vi "Auto-Write to Folder and file for FEC_YCC.vi"(0 "Current PD (mV)":dbl, 4 "Centering data?":bool, 5 "Record Mode \npath(1,2)":bool[](array[boolean]), 6 "data to be saved":dbl[][](array[numeric]) format="%0.2f", 7 "Who's Data":enum16{"YCC", "PYW", "LCH", "YYH"}(ring), 8 "File name add to the end \n(height)":string="h300", 9 "Save?":bool) -> (2 "Save to File Name":string, 3 "Save to Path":path)   [LabVIEW 2014]
uses:
  Main-Stage-PI/(Global) Current handle and LaserPower_YCC.vi
  <vilib>/Utility/file.llb/Write To Spreadsheet File (DBL).vi
panel:
  out "Folder name":string
  out "folder exists?":bool
  out "date/time string":string
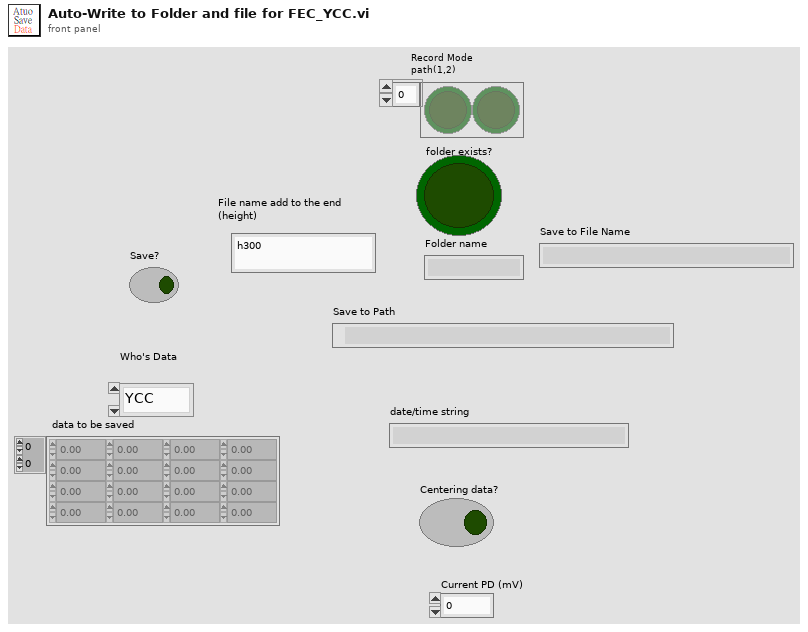
[diagram p1: front panel]
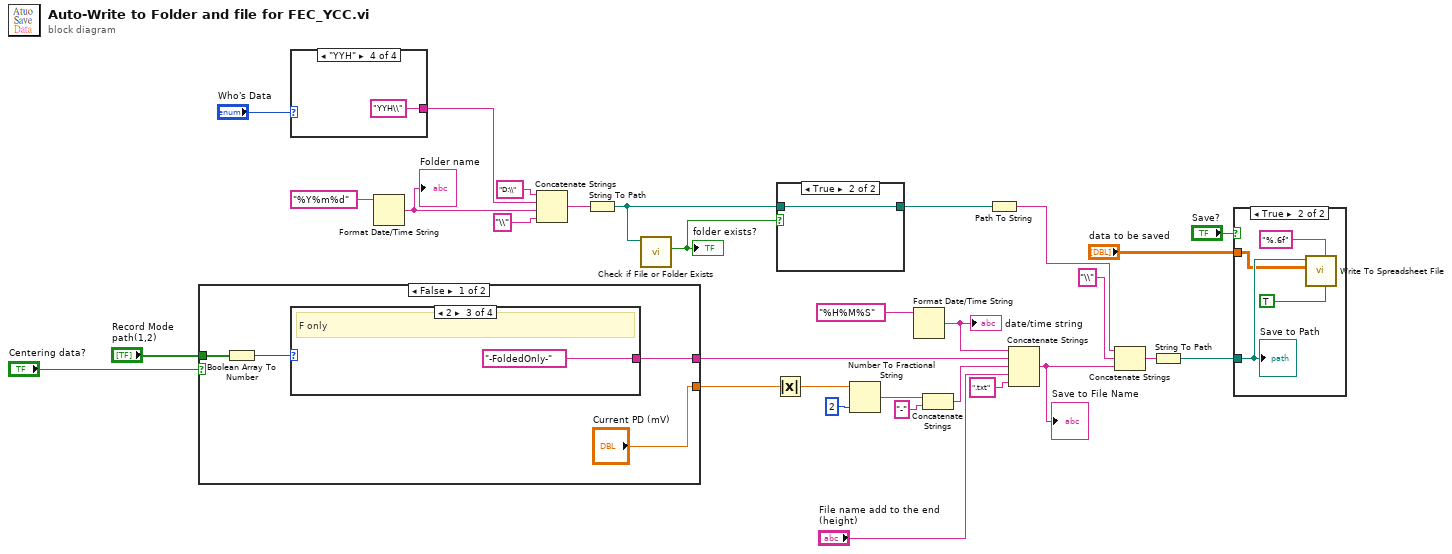
[diagram p0: block diagram]
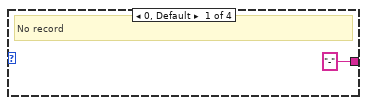
[diagram p2: hidden frame]
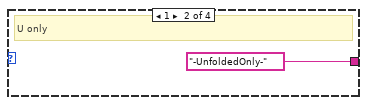
[diagram p3: hidden frame]
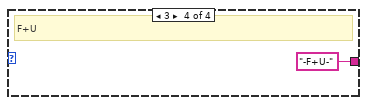
[diagram p4: hidden frame]
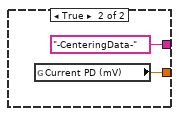
[diagram p5: hidden frame]
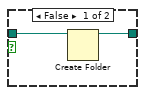
[diagram p6: hidden frame]
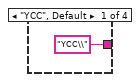
[diagram p8: hidden frame]
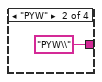
[diagram p9: hidden frame]
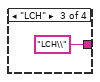
[diagram p10: hidden frame]
diagram:
  n1 = case shown="False" "Centering data?" {
    tunnel: "Record Mode \npath(1,2)" -> [w34 _]
    tunnel: [w32 "-CenteringData-" ("string")] -> w3
    tunnel: ["Current PD (mV)" w39] -> w1
    frame False {
      n2 = Boolean Array To Number(Boolean array=w34) -> (number=w33:u32)
      n3 = case shown="2" w33 {
        tunnel: ["-" ("string") "-UnfoldedOnly-" ("string") "-FoldedOnly-" ("string") "-F+U-" ("string")] -> w32
        frame 0, Default {
          # "No record"
        }
        frame 1 {
          # "U only"
        }
        frame 2 {
          # "F only"
        }
        frame 3 {
          # "F+U"
        }
      }
    }
    frame True {
      n4 = global read "(Global) Current handle and LaserPower_YCC.vi" "Current PD (mV)"() -> (w39:dbl)
    }
  }
  n5 = case shown="\"YYH\"" "Who's Data" {
    tunnel: ["YCC\\" ("string") "PYW\\" ("string") "LCH\\" ("string") "YYH\\" ("string")] -> w28
    frame "YCC", Default {
    }
    frame "PYW" {
    }
    frame "LCH" {
    }
    frame "YYH" {
    }
  }
  n6 = Format Date/Time String(time format string (%c)="%Y%m%d") -> (date/time string=w15:string)  [unwired: 2 in]
  "Folder name" <- w15
  n7 = Concatenate Strings("D:\\" ("string"), w28, w15, "\\" ("string")) -> (w27:string)
  n8 = String To Path(string=w27) -> (path=w18:path)
  n9 = call <vilib>:"Check if File or Folder Exists.vi"("path"=w18) -> ("file or folder exists?"=w17:bool)  [unwired: 8 in, 2 out]
  "folder exists?" <- w17
  n10 = Absolute Value(x=w1) -> (abs(x)=w2:dbl)
  n11 = case shown="True" w17 {
    tunnel: w18 -> [w46 w47]
    tunnel: [w45 w47] -> w23
    frame False {
      n12 = Create Folder(path (use dialog)=w46) -> (created path=w45:path)  [unwired: 2 in, 2 out]
    }
    frame True {
    }
  }
  n13 = Number To Fractional String(number=w2, precision (6)=i16 2) -> (F-format string=w8:string)  [unwired: 2 in]
  n14 = Format Date/Time String(time format string (%c)="%H%M%S") -> (date/time string=w12:string)  [unwired: 2 in]
  "date/time string" <- w12
  n15 = Concatenate Strings(w8, "-" ("string")) -> (w6:string)
  n16 = Path To String(path=w23) -> (string=w20:string)
  n17 = Concatenate Strings(w12, w3, w6, "File name add to the end \n(height)", ".txt" ("string")) -> (w14:string)
  "Save to File Name" <- w14
  n18 = Concatenate Strings(w20, "\\" ("string"), w14) -> (w22:string)
  n19 = String To Path(string=w22) -> (path=w21:path)
  n20 = case shown="True" "Save?" {
    tunnel: w21 -> [_ w50]
    tunnel: "data to be saved" -> [_ w49]
    frame False {
    }
    frame True {
      n21 = call-poly <vilib>:"Write To Spreadsheet File.vi"("transpose? (no:F)"=TRUE, "format (%.3f)"="%.6f", "2D data"=w49, "file path (dialog if empty)"=w50) -> ()  [unwired: 4 in, 1 out]
      "Save to Path" <- w50
    }
  }
